vi "加密解密字符串（XOR）应用举例.vi"() -> ()   [LabVIEW 2012]
panel:
  out "加密字符串":string
  out "输出字符串":string
  in  "密钥":u8=30
  in  "输入字符串":string
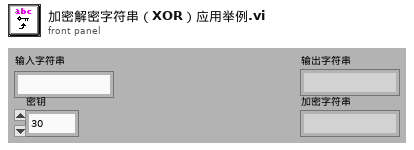
[diagram p1: front panel]
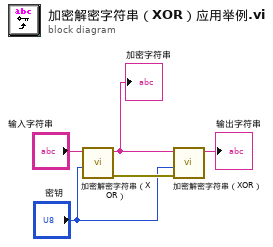
[diagram p0: block diagram]
diagram:
  n1 = call "加密解密字符串（XOR）.vi"("密钥"="密钥", "输入字符串"="输入字符串") -> ("error out"=w4:errorcluster, "输出字符串"=w2:string)  [unwired: 8 in]
  "加密字符串" <- w2
  n2 = call "加密解密字符串（XOR）.vi"("error in (no error)"=w4, "密钥"="密钥", "输入字符串"=w2) -> ("输出字符串"=→"输出字符串":string)  [unwired: 7 in, 1 out]
